vi "9211_Update Channels.vi"(8 "error in":errorcluster, 10 "Channels":T2(array[cluster]) {"Degree Range" items=["Raw Volts", "Degrees Kelvin", "Degrees Celsius", "Degrees Fahrenheit", "Degrees Rankine"]; "Thermocouple Type" items=["J", "K", "T", "E", "R", "S", "N", "B"]}, 11 "Node Ptr in":T1 format="%.0x") -> (0 "error out":errorcluster, 3 "Node Ptr out":T1 format="%.0x")   [LabVIEW 2017, in "Modules.lvlib" / "9211.lvclass"]
uses:
  9211.lvclass
  <vilib>/NI Veristand/Custom Device API/Custom Device Item Ref.ctl
  C:/Users/dbuck/Documents/GitHub/Scan-Engine-Custom-Device-Classes/Source/RSI Module/RSI Module.lvclass
  9211.lvclass/9211.ctl
  RSI Module/RSI Module.lvclass
  <vilib>/NI Veristand/Custom Device API/Custom Device API.lvlib
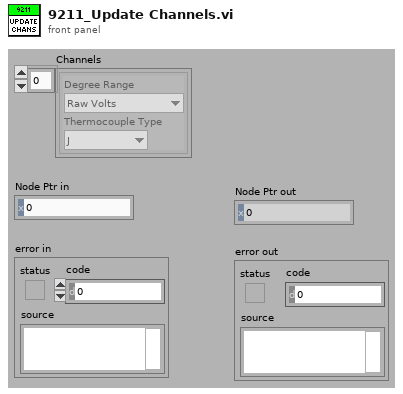
[diagram p1: front panel]
types:
  T1 = typedef "Custom Device API.lvlib/Custom Device Item Ref.ctl" = u64
  T2 = cluster{"Degree Range":u8, "Thermocouple Type":u8}[]
  T3 = typedef "Custom Device API.lvlib/Custom Device Channel.ctl" = cluster{"Type":T4, "Units":string, "Default Value":dbl, "Faultable":bool, "Scalable":bool}
  T4 = typedef "Custom Device API.lvlib/Custom Device Channel Type.ctl" = enum16{"Input", "Output"}
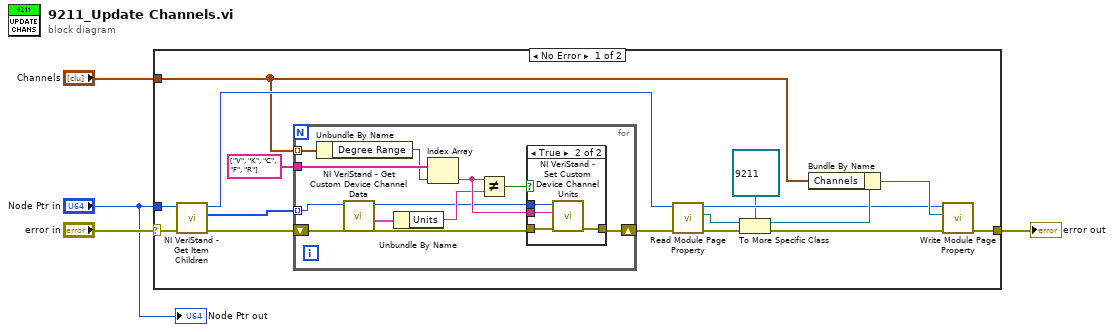
[diagram p0: block diagram]
diagram:
  n1 = case shown="No Error" "error in" {
    selector: "error in" -> [w11 w38]
    tunnel: [w18 w38] -> w4
    tunnel: "Node Ptr in" -> [w12 _]
    tunnel: "Channels" -> [w7 _]
    frame No Error {
      n2 = call <vilib>:"NI VeriStand - Get Item Children.vi"("error in (no error)"=w11, "Item Ref in"=w12) -> ("error out"=w8:errorcluster, "Child Refs"=w10:T1[], "Item Ref out"=w9:T1)  [unwired: 6 in, 1 out]
      n3 = for {
        tunnel: w10 -> [w22] mode=indexing
        shift-right: [w23] -> w5
        shift-left: w8 -> [w25]
        tunnel: w7 -> [w32] mode=indexing
        tunnel: string[] ["V", "K", "C", "F", "R"] -> [w31]
        n4 = Unbundle By Name(w32) -> ("Degree Range"=w30:u8)
        n5 = call <vilib>:"NI VeriStand - Get Custom Device Channel Data.vi"("error in (no error)"=w25, "Channel Ref in"=w22) -> ("error out"=w24:errorcluster, "Channel"=w27:T3, "Channel Ref out"=w21:T1)  [unwired: 4 in, 3 out]
        n6 = Unbundle By Name(w27) -> ("Units"=w26:string)
        n7 = Index Array(array=w31, index=w30) -> (element=w28:string)
        n8 = Not Equal?(x=w28, y=w26) -> (x != y?=w29:bool)
        n9 = case shown="True" w29 {
          tunnel: w21 -> [_ w37]
          tunnel: w28 -> [_ w36]
          tunnel: w24 -> [w33 w35]
          tunnel: [w33 w34] -> w23
          frame False {
          }
          frame True {
            n10 = call <vilib>:"NI VeriStand - Set Custom Device Channel Units.vi"("error in (no error)"=w35, "Units"=w36, "Channel Ref in"=w37) -> ("error out"=w34:errorcluster)  [unwired: 7 in, 1 out]
          }
        }
      }
      n11 = call "Read Module Page Property.vi"("error in (no error)"=w5, "Node Ptr In"=w9) -> ("error out"=w15:errorcluster, "RSI Module"=w14:refnum<class "RSI Module.lvclass">, "Node Ptr Out"=w17:T1)  [unwired: 7 in]
      n12 = To More Specific Class(target class=refnum<class "9211.lvclass"> refnum ("9205 in"), reference=w14, error in=w15) -> (specific class reference=w19:refnum<class "9211.lvclass">, error out=w16:errorcluster)
      n13 = Bundle By Name(cluster=w19, "Channels"=w7) -> (w20:refnum<class "9211.lvclass">)
      n14 = call "Write Module Page Property.vi"("error in (no error)"=w16, "RSI Module"=w20, "Node Ptr In"=w17) -> ("error out"=w18:errorcluster)  [unwired: 6 in, 2 out]
    }
    frame Error {
    }
  }
  "error out" <- w4
  "Node Ptr out" <- "Node Ptr in"
